vi "Config MotionSystem.vi"(8 "error in (no error)":errorcluster, 11 "Configuration in":refnum<class "Configuration.lvclass">) -> (0 "error out":errorcluster, 3 "Configuration out":refnum<class "Configuration.lvclass">)   [LabVIEW 2016, in "MotionSystem.lvlib" / "MotionSystem Configuration.lvclass"]
uses:
  <userlib>/Common Components/Hardware/Abstract System/MotionSystem/MotionSystem Config/MotionSystem Configuration.lvclass
  <userlib>/Configuration Dialog Actor/Configuration.lvclass
  <userlib>/Common Components/Hardware/Abstract System/MotionSystem/MotionSystem Config/RxRyZ Limits.ctl
  C:/Program Files (x86)/National Instruments/LabVIEW 2016/user.lib/Configuration Dialog Actor/Configuration.lvclass
  C:/Program Files (x86)/National Instruments/LabVIEW 2016/vi.lib/ActorFramework/Actor/Actor.lvclass
  <vilib>/ActorFramework/Actor/Actor.lvclass/Actor.ctl
  <userlib>/Common Components/Hardware/Abstract System/MotionSystem/MotionSystem Config/MotionSystem Configuration.lvclass/MotionSystem Configuration.ctl
  <vilib>/ActorFramework/Actor/Actor.lvclass
panel:
  in  "RxRyZ limits":T1 caption="Rx, Ry, Z limits" {"Z (um)"."soft limit max" format="%#_6f um"; "Z (um)"."soft limit min" format="%#_6f um"; "Ry (deg)"."soft limit max" format="%#_6f deg"; "Ry (deg)"."soft limit min" format="%#_6f deg"; "Rx (deg)"."soft limit max" format="%#_6f deg"; "Rx (deg)"."soft limit min" format="%#_6f deg"}
  in  "Revert":bool
  in  "Apply":bool
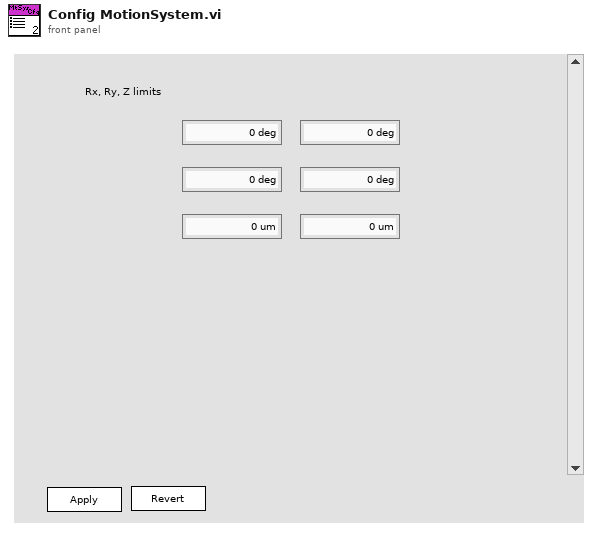
[diagram p1: front panel]
types:
  T1 = typedef "MotionSystem.lvlib/MotionSystem Configuration.lvclass/RxRyZ Limits.ctl" = cluster{"Rx (deg)":cluster{"label":string, "soft limit min":dbl, "soft limit max":dbl}, "Ry (deg)":cluster{"label":string, "soft limit min":dbl, "soft limit max":dbl}, "Z (um)":cluster{"label":string, "soft limit min":dbl, "soft limit max":dbl}}
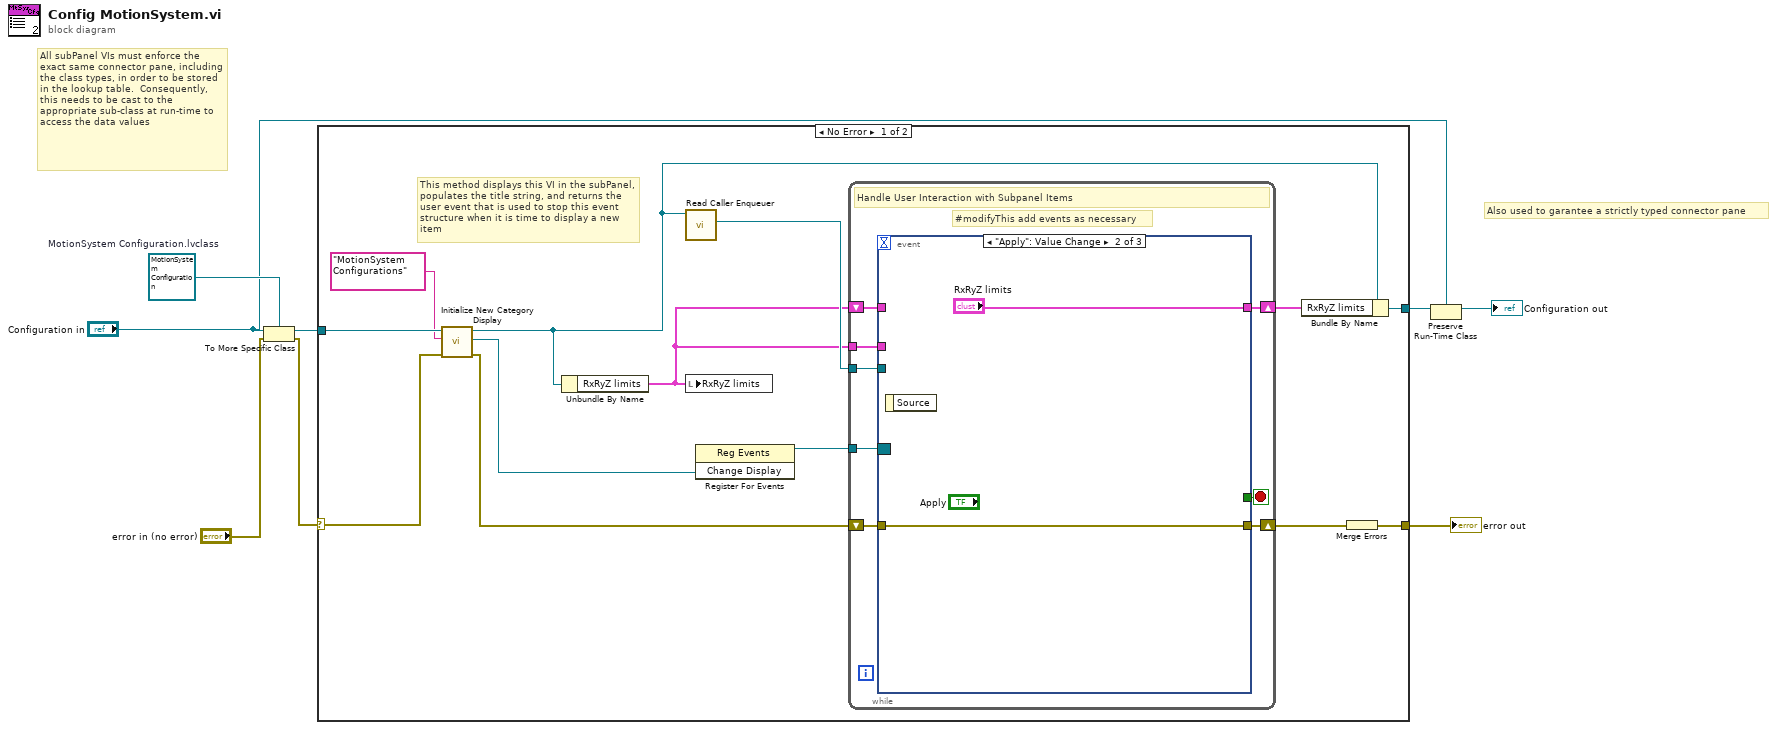
[diagram p0: block diagram]
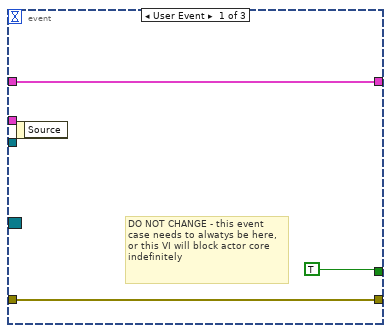
[diagram p2: hidden frame]
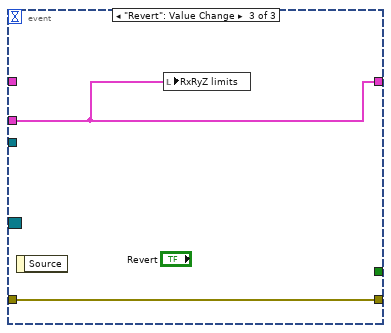
[diagram p3: hidden frame]
diagram:
  w5 = refnum<class "MotionSystem Configuration.lvclass"> refnum  # MotionSystem Configuration.lvclass
  # "Also used to garantee a strictly typed connector pane"
  # "All subPanel VIs must enforce the exact same connector pane, including the class types, in order to be stored in the lookup table.  Consequently, this needs to be cast to the appropriate sub-class at run-time to access the data values"
  n1 = To More Specific Class(target class=w5, reference="Configuration in", error in="error in (no error)") -> (specific class reference=w6:refnum<class "MotionSystem Configuration.lvclass">, error out=w1:errorcluster)
  n2 = case shown="No Error" w1 {
    selector: w1 -> [w14 w37]
    tunnel: w6 -> [w21 w38]
    tunnel: [w10 w38] -> w8
    tunnel: [w20 w37] -> w7
    frame No Error {
      # "This method displays this VI in the subPanel, populates the title string, and returns the user event that is used to stop this event structure when it is time to display a new item"
      n3 = call <userlib>:"Initialize New Category Display.vi"("error in (no error)"=w14, "Name to Display"="MotionSystem Configurations", "Configuration in"=w21) -> ("error out"=w15:errorcluster, "Change Display"=w18:refnum<user-event>, "Configuration Out"=w12:refnum<class "MotionSystem Configuration.lvclass">)  [unwired: 6 in]
      n4 = Unbundle By Name(w12) -> ("RxRyZ limits"=w11:T1)
      n5 = call <vilib>:"Read Caller Enqueuer.vi"("Actor"=w12) -> ("Caller Enqueuer"=w13:refnum<class "Message Enqueuer.lvclass">)  [unwired: 10 in]
      n6 = local write "RxRyZ limits"(w11) -> ()
      n7 = register-events(w18) -> (reference out=w17:refnum<event-registration>)  [unwired: 2 in, 1 out]
      n8 = while {
        tunnel: w17 -> [w28]
        shift-right: [w27] -> w16
        shift-left: w15 -> [w26]
        shift-right: [w24] -> w9
        shift-left: w11 -> [w25]
        tunnel: w11 -> [w23]
        tunnel: w13 -> [w22]
        stop <- w29 stop-if-true
        # "#modifyThis add events as necessary"
        # "Handle User Interaction with Subpanel Items"
        n9 = event shown="[1] \"Apply\": Value Change" {
          selector: w28 -> [_ _ _]
          dyn-events: _ -> [_ _ _]
          timeout: _ -> [_ _ _]
          tunnel: [TRUE _ _] -> w29
          tunnel: [w32 w34 w36] -> w27
          tunnel: w26 -> [w32 w34 w36]
          tunnel: w25 -> [w31 _ _]
          tunnel: [w31 "RxRyZ limits" w35] -> w24
          tunnel: w23 -> [_ _ w35]
          tunnel: w22 -> [_ _ _]
          event User Event {
            # "DO NOT CHANGE - this event case needs to alwatys be here, or this VI will block actor core indefinitely"
            n10 = event-data() -> ()  [unwired: 1 in, 1 out]
          }
          event "Apply": Value Change {
            n11 = event-data() -> ()  [unwired: 1 in, 1 out]
          }
          event "Revert": Value Change {
            n12 = event-data() -> ()  [unwired: 1 in, 1 out]
            n13 = local write "RxRyZ limits"(w35) -> ()
          }
        }
      }
      n14 = Bundle By Name(cluster=w12, "RxRyZ limits"=w9) -> (w10:refnum<class "MotionSystem Configuration.lvclass">)
      n15 = Merge Errors(w16) -> (w20:errorcluster)
    }
    frame Error {
    }
  }
  "error out" <- w7
  n16 = Preserve Run-Time Class(object in=w8, 2:"Configuration in") -> (object out=→"Configuration out":refnum<class "Configuration.lvclass">)  [unwired: 1 in, 1 out]
